vi "FP to PGSQL.vi"(4 "Mode":u16, 6 "Status Array":u32[](array[numeric]), 8 "PT Data":dbl[](array[numeric]), 9 "MG Data":dbl[](array[numeric]), 10 "FP Data":sgl[](array[numeric]), 11 "Inst.FP":refnum<class "Inst.FP.lvclass">) -> (2 "GetAll":T1, 3 "Inst.FP out":refnum<class "Inst.FP.lvclass">)   [LabVIEW 2019, in "Inst.FP.lvclass"]
uses:
  Inst.FP.lvclass
  Typedefs/Inst.FP.getAll--Cluster.ctl
  <userlib>/LevyLab/Instrument Framework/Instrument/Instrument.lvclass
  C:/Program Files (x86)/National Instruments/LabVIEW 2019/user.lib/LevyLab/Instrument Framework/Instrument Types/Cryostat/Instrument.Cryostat.lvclass
  C:/Program Files (x86)/National Instruments/LabVIEW 2019/user.lib/LevyLab/Instrument Framework/Instrument/Instrument.lvclass
  C:/Program Files (x86)/National Instruments/LabVIEW 2019/vi.lib/JKI/JKI SMO/SMO/SMO.lvclass
  FP-TC-Shared/FP-TC-Shared.lvclass
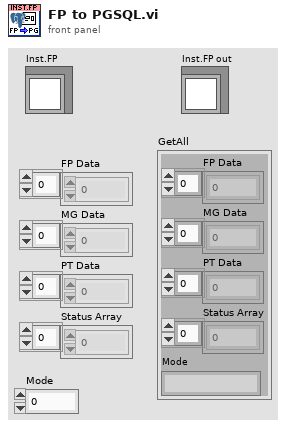
[diagram p1: front panel]
types:
  T1 = typedef "Inst.FP.lvclass/Inst.FP.getAll--Cluster.ctl" = cluster{"FP Data":dbl[], "MG Data":dbl[], "PT Data":dbl[], "Status Array":u32[], "Mode":string}
  T2 = typedef "Inst.FP.lvclass/Inst.FP.Type--Enum.ctl" = enum32{"Wet", "CF"}
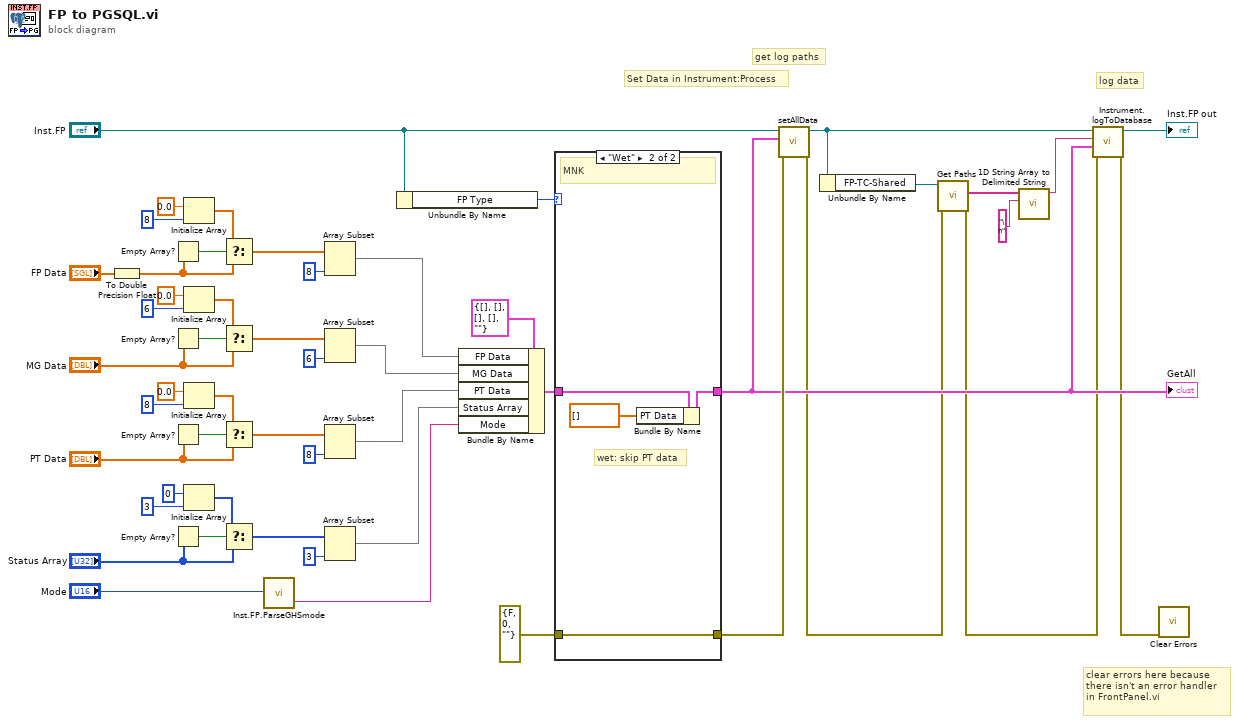
[diagram p0: block diagram]
diagram:
  # "log data"
  # "get log paths"
  # "clear errors here because there isn't an error handler in FrontPanel.vi"
  # "Set Data in Instrument:Process"
  n1 = To Double Precision Float(number="FP Data") -> (double precision float=w14:dbl[])
  n2 = Empty Array?(array=w14) -> (empty?=w34:bool)
  n3 = Empty Array?(array="MG Data") -> (empty?=w28:bool)
  n4 = Empty Array?(array="PT Data") -> (empty?=w19:bool)
  n5 = Empty Array?(array="Status Array") -> (empty?=w25:bool)
  n6 = Initialize Array(0.0 ("element"), 8 ("dimension size")) -> (w33:dbl[])
  n7 = Initialize Array(0.0 ("element"), 6 ("dimension size")) -> (w16:dbl[])
  n8 = Initialize Array(0.0 ("element"), 8 ("dimension size")) -> (w15:dbl[])
  n9 = Initialize Array(u32 0 ("element"), 3 ("dimension size")) -> (w26:u32[])
  n10 = Select(t=w33, s=w34, f=w14) -> (s? t:f=w31:dbl[])
  n11 = Select(t=w16, s=w28, f="MG Data") -> (s? t:f=w27:dbl[])
  n12 = Select(t=w15, s=w19, f="PT Data") -> (s? t:f=w18:dbl[])
  n13 = Select(t=w26, s=w25, f="Status Array") -> (s? t:f=w22:u32[])
  n14 = call "Inst.FP.ParseGHSmode.vi"("GHS.Mode"="Mode") -> ("mode string"=w43:string)  [unwired: 1 in, 1 out]
  n15 = Array Subset(array=w31, length=8) -> (w42:dbl[])  [unwired: 1 in]
  n16 = Array Subset(array=w27, length=6) -> (w39:dbl[])  [unwired: 1 in]
  n17 = Array Subset(array=w18, length=8) -> (w17:dbl[])  [unwired: 1 in]
  n18 = Array Subset(array=w22, length=3) -> (w37:u32[])  [unwired: 1 in]
  n19 = Unbundle By Name("Inst.FP") -> ("FP Type"=w12:T2)
  n20 = Bundle By Name(cluster=T1 {"FP Data"=[], "MG Data"=[], "PT Data"=[], "Status Array"=[], "Mode"=""} ("GetAll"), "FP Data"=w42, "MG Data"=w39, "PT Data"=w17, "Status Array"=w37, "Mode"=w43) -> (w41:T1)
  n21 = case shown="\"Wet\"" w12 {
    tunnel: errorcluster {"status"=FALSE, "code"=0, "source"=""} ("error in (no error)") -> [w53 w57]
    tunnel: [w53 w57] -> w13
    tunnel: w41 -> [w52 w55]
    tunnel: [w52 w56] -> w9
    frame "CF" {
      # "CF"
    }
    frame "Wet" {
      # "wet: skip PT data"
      # "MNK"
      n22 = Bundle By Name(cluster=w55, "PT Data"=dbl[] []) -> (w56:T1)
    }
  }
  "GetAll" <- w9
  n23 = call <userlib>:"setAllData.vi"("error in (no error)"=w13, "AllData"=w9, "Instrument in"="Inst.FP") -> ("error out"=w3:errorcluster, "Instrument out"=w4:refnum<class "Inst.FP.lvclass">)  [unwired: 7 in]
  n24 = Unbundle By Name(w4) -> ("FP-TC-Shared"=w7:refnum<class "FP-TC-Shared.lvclass">)
  n25 = call-dynamic "Get Paths.vi"("error in (no error)"=w3, "FP-TC-Shared in"=w7) -> ("error out"=w2:errorcluster, "Paths"=w6:string[])  [unwired: 7 in, 1 out]
  n26 = call <vilib>:"1D String Array to Delimited String.vi"("delimiter"="\n", "string array"=w6) -> ("delimited string"=w1:string)  [unwired: 9 in]
  n27 = call <userlib>:"Instrument.logToDatabase.vi"("error in (no error)"=w2, "Data"=w9, "Paths"=w1, "Instrument"=w4) -> ("error out"=w8:errorcluster, "Instrument out"=→"Inst.FP out":refnum<class "Inst.FP.lvclass">)  [unwired: 6 in]
  n28 = call <vilib>:"Clear Errors.vi"("error in (no error)"=w8) -> ()  [unwired: 5 in, 2 out]
